vi "MakeCalFileList.vi"(0 "Calibration Folder Path":path=path "M:/Preferences/Rig_Setups/All_Rigs/Calibrations/5HoleProbe", 1 "Old5HoleProbe?":bool, 2 "Probe Type":u16(ring)=5 items=["5-Hole Probe"=5, "OmniProbe"=12]) -> (3 "MultiProbeCals":string caption="DelimitedCalFileList (for MultiProbe)", 4 "AeroFlowCals":path[](array[path]) caption="Calibration File Array (for AeroFlow)")   [LabVIEW 2021]
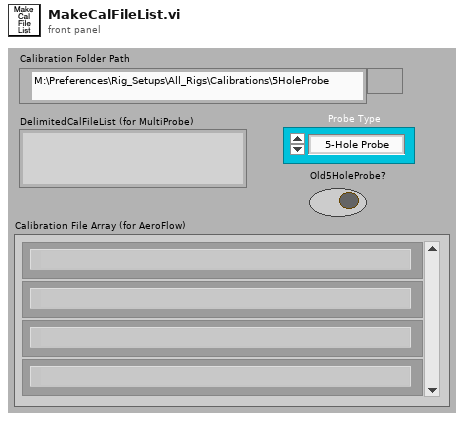
[diagram p1: front panel]
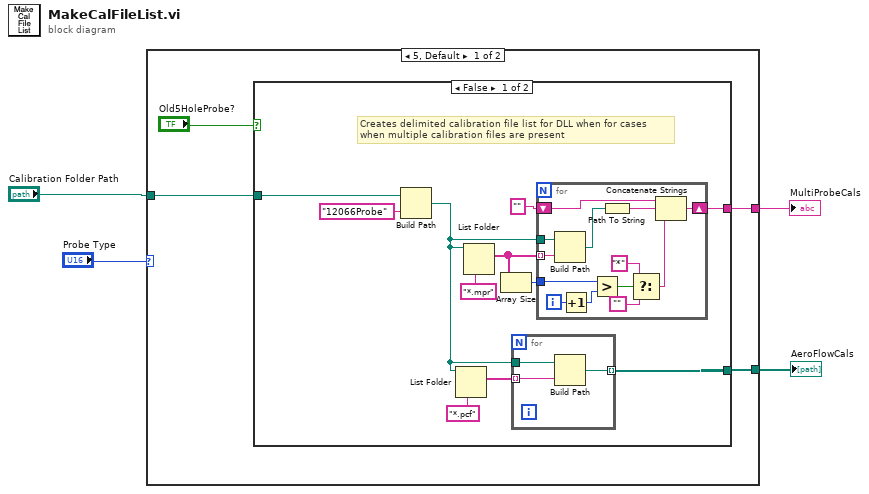
[diagram p0: block diagram]
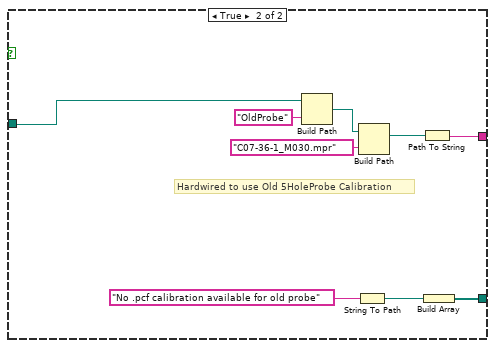
[diagram p2: hidden frame]
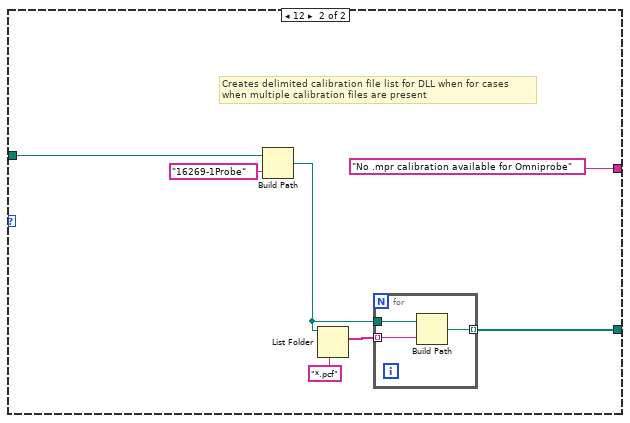
[diagram p3: hidden frame]
diagram:
  n1 = case shown="5, Default" "Probe Type" {
    tunnel: "Calibration Folder Path" -> [w8 w51]
    tunnel: [w7 w50] -> w3
    tunnel: [w6 "No .mpr calibration available for Omniprobe" ("name or relative path")] -> w2
    frame 5, Default {
      n2 = case shown="False" "Old5HoleProbe?" {
        tunnel: w8 -> [w19 w43]
        tunnel: [w15 w39] -> w7
        tunnel: [w13 w36] -> w6
        frame False {
          # "Creates delimited calibration file list for DLL when for cases\nwhen multiple calibration files are present"
          n3 = Build Path(base path=w19, name or relative path="12066Probe") -> (appended path=w14:path)
          n4 = List Folder(path=w14, pattern="*.pcf") -> (filenames=w16:string[])  [unwired: 2 in, 3 out]
          n5 = List Folder(path=w14, pattern="*.mpr") -> (filenames=w10:string[])  [unwired: 2 in, 3 out]
          n6 = Array Size(array=w10) -> (size(s)=w9:i32)
          n7 = for {
            tunnel: w14 -> [w35]
            tunnel: w16 -> [w34] mode=indexing
            tunnel: [w33] -> w15 mode=indexing
            n8 = Build Path(base path=w35, name or relative path=w34) -> (appended path=w33:path)
          }
          n9 = for {
            tunnel: w14 -> [w32]
            tunnel: w10 -> [w31] mode=indexing
            shift-right: [w27] -> w13
            shift-left: "" -> [w28]
            tunnel: w9 -> [w25]
            i -> [w26]
            n10 = Build Path(base path=w32, name or relative path=w31) -> (appended path=w30:path)
            n11 = Increment(x=w26) -> (x+1=w20:i32)
            n12 = Greater?(x=w25, y=w20) -> (0:w24:bool)
            n13 = Path To String(path=w30) -> (string=w29:string)
            n14 = Select(t="*", s=w24, f="") -> (s? t:f=w22:string)
            n15 = Concatenate Strings(w28, w29, w22) -> (w27:string)
          }
        }
        frame True {
          # "Hardwired to use Old 5HoleProbe Calibration"
          n16 = Build Path(base path=w43, name or relative path="OldProbe") -> (appended path=w41:path)
          n17 = String To Path(string="No .pcf calibration available for old probe" ("name or relative path")) -> (path=w37:path)
          n18 = Build Path(base path=w41, name or relative path="C07-36-1_M030.mpr") -> (appended path=w40:path)
          n19 = Path To String(path=w40) -> (string=w36:string)
          n20 = Build Array(w37) -> (w39:path[])
        }
      }
    }
    frame 12 {
      # "Creates delimited calibration file list for DLL when for cases\nwhen multiple calibration files are present"
      n21 = Build Path(base path=w51, name or relative path="16269-1Probe") -> (appended path=w46:path)
      n22 = List Folder(path=w46, pattern="*.pcf") -> (filenames=w47:string[])  [unwired: 2 in, 3 out]
      n23 = for {
        tunnel: w46 -> [w54]
        tunnel: w47 -> [w53] mode=indexing
        tunnel: [w52] -> w50 mode=indexing
        n24 = Build Path(base path=w54, name or relative path=w53) -> (appended path=w52:path)
      }
    }
  }
  "MultiProbeCals" <- w2
  "AeroFlowCals" <- w3
